vi "configure.vi"(8 "error in (no error)":errorcluster, 9 "Value":i32, 10 "ILC":refnum<class "ILC.lvclass">, 11 "ConfigureILCSSRStrategy in":refnum<class "ConfigureILCSSRStrategy.lvclass">) -> (0 "error out":errorcluster, 2 "ILC 2":refnum<class "ILC.lvclass">, 3 "ConfigureILCSSRStrategy out":refnum<class "ConfigureILCSSRStrategy.lvclass">)   [LabVIEW 2016, in "ConfigureILCSSRStrategy.lvclass"]
uses:
  ConfigureILCSSRStrategy.lvclass
  Common_ILC/ILC/ILC.lvclass
  Common_ILC/ILC/ILC.lvclass/ILC.ctl
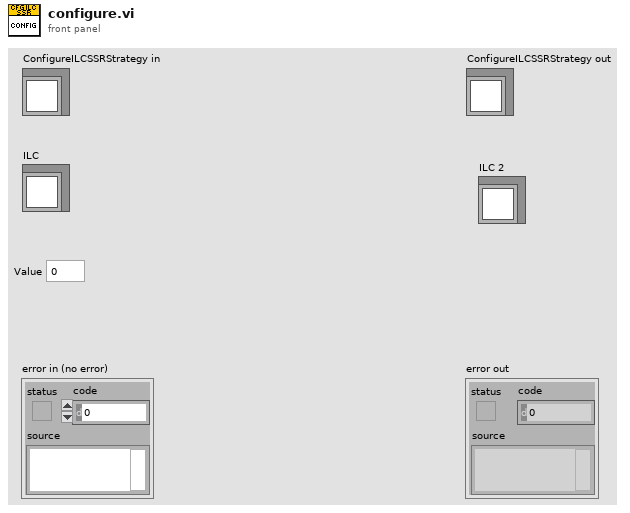
[diagram p1: front panel]
types:
  T1 = typedef "ILCCommon.lvlib/ILCTypedefs.lvlib/Outputs.ctl" = cluster{"Step & Direction":i16, "Blower RPM":u8, "PWM (SSR)":u8, "Ch1":u16, "Ch2":u16, "Ch3":u16, "Ch4":u16}
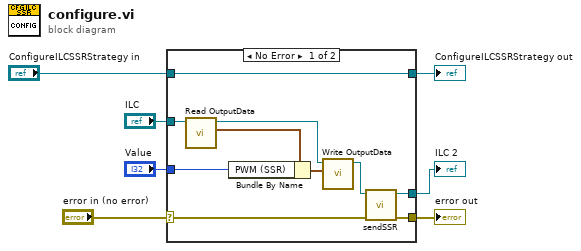
[diagram p0: block diagram]
diagram:
  n1 = case shown="No Error" "error in (no error)" {
    selector: "error in (no error)" -> [w10 w20]
    tunnel: [w9 w20] -> w6
    tunnel: [w17 w19] -> w4
    tunnel: "ConfigureILCSSRStrategy in" -> [w17 w19]
    tunnel: "ILC" -> [w8 w18]
    tunnel: "Value" -> [w13 _]
    tunnel: [w11 w18] -> w1
    frame No Error {
      n2 = call "Read OutputData.vi"("ILC in"=w8) -> ("OutputData"=w16:T1, "ILC out"=w14:refnum<class "ILC.lvclass">)  [unwired: 9 in]
      n3 = Bundle By Name(cluster=w16, "PWM (SSR)"=w13) -> (w15:T1)
      n4 = call "Write OutputData.vi"("OutputData"=w15, "ILC in"=w14) -> ("ILC out"=w12:refnum<class "ILC.lvclass">)  [unwired: 9 in]
      n5 = call "sendSSR.vi"("error in (no error)"=w10, "ILC in"=w12) -> ("error out"=w9:errorcluster, "ILC out"=w11:refnum<class "ILC.lvclass">)  [unwired: 8 in]
    }
    frame Error {
    }
  }
  "error out" <- w6
  "ConfigureILCSSRStrategy out" <- w4
  "ILC 2" <- w1
